vi "Evaluate Destination Subpanel.vi"(9 "Destination Subpanel":T1, 11 "Viewable in":refnum<class "IViewable.lvclass">) -> (2 "Already Inserted?":bool)   [LabVIEW 2015, in "IViewable.lvlib" / "IViewable.lvclass"]
uses:
  IViewable.lvclass
  ProtectedSubpanel/Protected Subpanel Reference.ctl
  ProtectedSubpanel/ProtectedSubpanel.lvclass
  IViewable.lvclass/IViewable.ctl
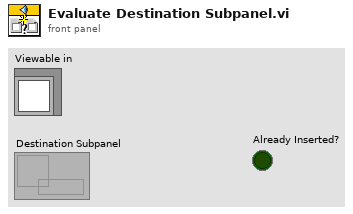
[diagram p1: front panel]
types:
  T1 = typedef "IViewable.lvlib/ProtectedSubpanel.lvclass/Protected Subpanel Reference.ctl" = refnum<data-value>
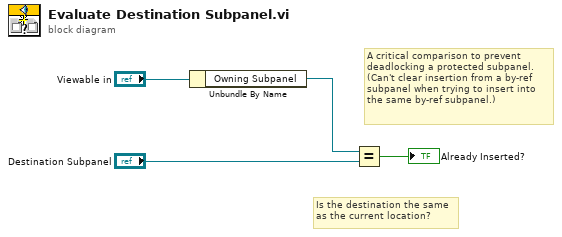
[diagram p0: block diagram]
diagram:
  # "Is the destination the same\nas the current location?"
  # "A critical comparison to prevent\ndeadlocking a protected subpanel. \n(Can't clear insertion from a by-ref\nsubpanel when trying to insert into\nthe same by-ref subpanel.)"
  n1 = Unbundle By Name("Viewable in") -> ("Owning Subpanel"=w3:T1)
  n2 = Equal?(x=w3, y="Destination Subpanel") -> (x = y?=→"Already Inserted?":bool)
